vi "Main.vi"() -> ()   [LabVIEW 2011]
uses:
  2-Think/2 Typedefs/Which Boat.ctl
  0x2-OCU-Think Comm/0x2 Typedefs/Waypoints List.ctl
  2-Think/2 Classes/Waypoint/Waypoint.lvclass
  0x2-OCU-Think Comm/0x2 Typedefs/Current Waypoint.ctl
  2-Think/2 Typedefs/eStopCommand.ctl
  0x2-OCU-Think Comm/0x2 Typedefs/ocuMessage.ctl
  0x2-OCU-Think Comm/0x2 Typedefs/ocuCommands.ctl
  <vilib>/Platform/TimedLoop/XDataNode/timing_clust.ctl
  <vilib>/Platform/TimedLoop/XDataNode/nitl_modes.ctl
  <vilib>/Platform/TimedLoop/XDataNode/wakeup.ctl
  <vilib>/vision/Image Controls.llb/IMAQ Image.ctl
  2-Think/2 Globals/2 Global.vi
  2-Think/2 Globals/2 Message Logger.vi
  <vilib>/Platform/TimedLoop/XDataNode/XDataNode.xnode
  <vilib>/Platform/TimedLoop/XDataNode/XDNodeRunTimeDep.lvlib
  0x2-OCU-Think Comm/0x2 Classes/NetworkStreams/Writer/NetworkStreamWriter.lvclass
  0x2-OCU-Think Comm/0x2 Classes/NetworkStreams/Reader/NetworkStreamReader.lvclass
  2-Think/2 Classes/Logger/Logger.lvclass
panel:
  in  "Enable logging?":bool
  in  "Data storage folder":path
  in  "Which Boat Am I?":T1=enum."Simulation"
  out "E-stop freq.":dbl
  out "Act freq.":dbl
  out "Sense freq.":dbl
  out "Think freq.":dbl
  in  "E-Stop":bool
  # "this is the parent VI under which \nSense Think and Act run."
  # "Will save to U:\\Logs when run on the RIO"
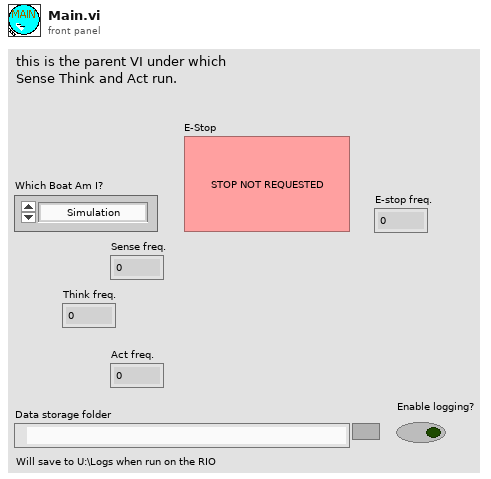
[diagram p1: front panel]
types:
  T1 = typedef "Which Boat.ctl" = enum16{"Competition Boat", "Small RC", "Simulation"}
  T2 = typedef "Waypoints List.ctl" = refnum<class "Waypoint.lvclass">[]
  T3 = typedef "Current Waypoint.ctl" = i32
  T4 = typedef "eStopCommand.ctl" = enum16{"Reset E-Stop", "Get E-Stop", "Set E-Stop"}
  T5 = typedef "ocuMessage.ctl" = cluster{"OCU Command":T6, "Data":variant}
  T6 = typedef "ocuCommands.ctl" = enum16{"Pass", "Send override", "Add waypoint", "Delete waypoint", "Set waypoint number", "Stop", "Add Mission"}
  T7 = typedef "XDNodeRunTimeDep.lvlib/timing_clust.ctl" = cluster{"Expected End [f-1]":u64, "Actual End [f-1]":u64, "Finished Late? [f-1]":bool, "Expected End [i-1]":u64, "Actual End [i-1]":u64, "Finished Late? [i-1]":bool, "Expected Start [i]":u64, "Actual Start [i]":u64, "Expected Start [f]":u64, "Actual Start [f]":u64, "Source Name":string, "Structure Name":string, "Period":i64, "Deadline":i64, "Offset":i64, "Start":i64, "Priority":i32, "Timeout":i32, "Mode":T8, "Wakeup Reason":T9, "Error":errorcluster, "Source Type":string, "Secondary Source Type":string, "Global End Time":u64, "Global Start Time":u64, "Frame Duration":u64, "Iteration Duration":u64, "Assigned CPU":i32, "I/O Scan Engine Mode":u32}
  T8 = typedef "XDNodeRunTimeDep.lvlib/nitl_modes.ctl" = enum32{"No Change", "Process missed periods, maintain original phase", "Discard missed periods, maintain original phase", "Process missed periods, ignore original phase", "Discard missed periods, ignore original phase"}
  T9 = typedef "XDNodeRunTimeDep.lvlib/wakeup.ctl" = enum32{"Normal", "Aborted", "Asynchronous wakeup", "Timing source error", "Timed loop error", "Timeout"}
  T10 = typedef "IMAQ Image.ctl" = refnum<image>
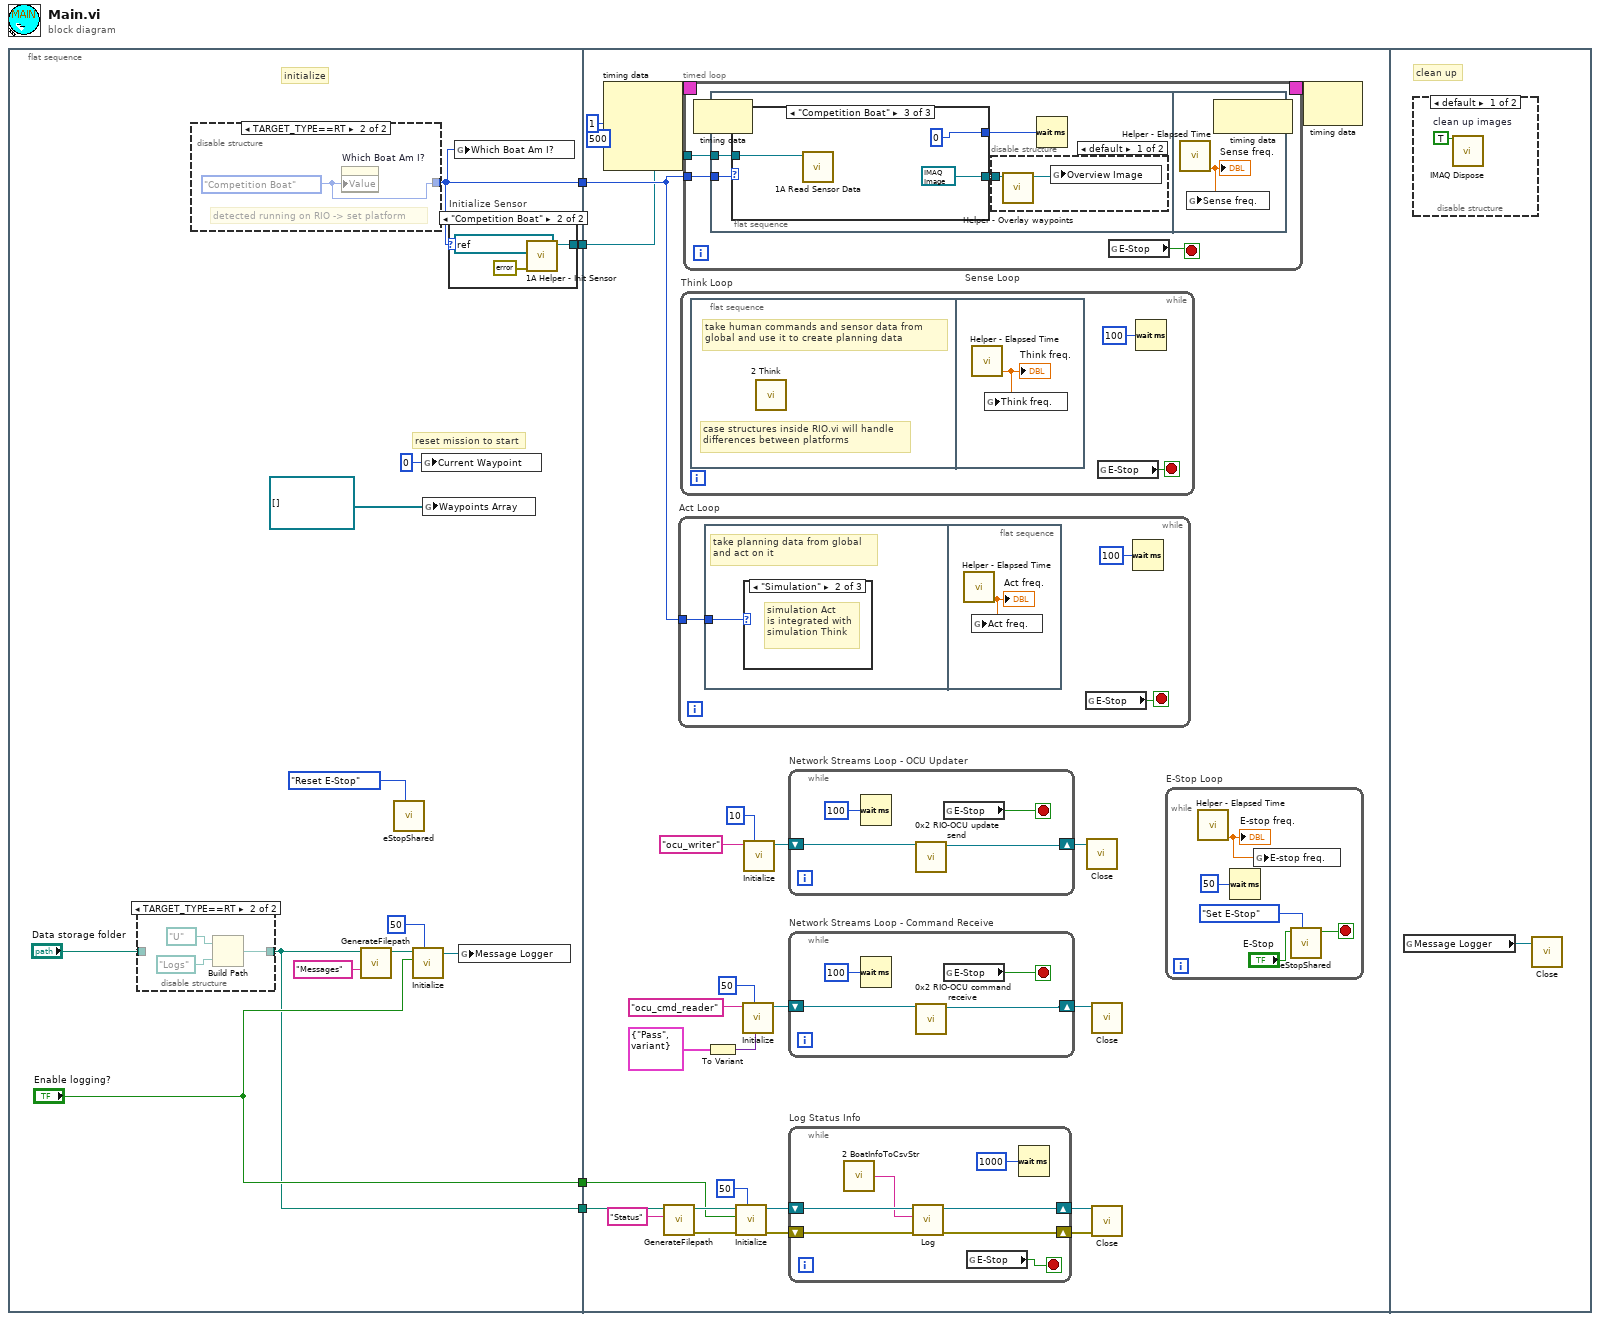
[diagram p0: block diagram]
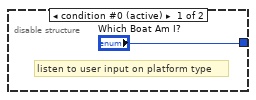
[diagram p4: hidden frame]
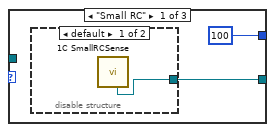
[diagram p6: hidden frame]
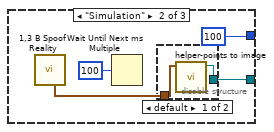
[diagram p8: hidden frame]
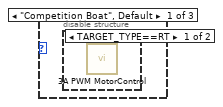
[diagram p10: hidden frame]
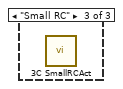
[diagram p12: hidden frame]
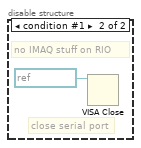
[diagram p13: hidden frame]
diagram:
  n1 = flat-sequence {
    tunnel: [w13] -> w4
    tunnel: [w14] -> w3
    tunnel: [w6] -> w2
    tunnel: ["Enable logging?"] -> w1
    tunnel: w4 -> [w51]
    tunnel: w3 -> [w50]
    tunnel: w2 -> [w30]
    tunnel: w1 -> [w26]
    frame #0 {
      # "reset mission to start"
      # "initialize"
      n2 = disable-structure shown="TARGET_TYPE==RT" {
        disable-tunnel: "Data storage folder" -> [w17 _]
        disable-tunnel: [w17 w18] -> w6
        frame condition #0 (active) {
        }
        frame condition #1 {
          n3 = Build Path(base path=path "U:/" ("Data storage folder"), name or relative path=path "Logs" ("Data storage folder")) -> (appended path=w18:path)
        }
      }
      n4 = disable-structure shown="TARGET_TYPE==RT" {
        disable-tunnel: ["Which Boat Am I?" w25] -> w13
        frame condition #0 (active) {
          # "listen to user input on platform type"
        }
        frame condition #1 {
          w25 = Which_Boat."Competition Boat" ("Which Boat Am I?")
          # "detected running on RIO -> set platform"
          n5 = property on="Which Boat Am I?" class="Enum (strict)"("Value"=w25) -> ()  [unwired: 2 in, 2 out]
        }
      }
      n6 = call "GenerateFilepath.vi"("Identifier"="Messages", "Data storage folder"=w6) -> ("File path out"=w9:path)  [unwired: 8 in, 1 out]
      n7 = call "eStopShared.vi"("Command"=eStopCommand."Reset E-Stop") -> ()  [unwired: 9 in, 2 out]
      n8 = call "Initialize.vi"("buffer size"=50, "Enable? (T)"="Enable logging?", "File path"=w9) -> ("Logger out"=w10:refnum<class "Logger.lvclass">)  [unwired: 7 in, 1 out]
      n9 = global write "2 Global.vi" "Current Waypoint"(T3 0 ("Current Waypoint")) -> ()
      n10 = global write "2 Global.vi" "Waypoints Array"(T2 [] ("Waypoints Array")) -> ()
      n11 = case "Initialize Sensor" shown="\"Competition Boat\"" w13 {
        tunnel: [_ w21] -> w14
        frame Default {
        }
        frame "Competition Boat" {
          n12 = call "1A Helper - Init Sensor.vi"("error in (no error)"=errorcluster {"status"=FALSE, "code"=0, "source"=""}, "VISA Refnum in"=refnum<visa-resource-name> "ASRL1::INSTR" ("VISA resource name")) -> ("VISA Refnum out"=w21:refnum<visa-resource-name>)  [unwired: 7 in, 2 out]
        }
      }
      n13 = global write "2 Global.vi" "Which Boat Am I?"(w13) -> ()
      n14 = global write "2 Message Logger.vi" "Message Logger"(w10) -> ()
    }
    frame #1 {
      n15 = node-c288(i64 1 ("Period"), 500 ("Priority")) -> (w49:T7)  [unwired: 2 in]
      n16 = call "GenerateFilepath.vi"("Identifier"="Status", "Data storage folder"=w30) -> ("error out"=w34:errorcluster, "File path out"=w35:path)  [unwired: 8 in]
      n17 = while "Act Loop" {
        tunnel: w51 -> [w105]
        stop <- w106 stop-if-true
        n18 = flat-sequence {
          tunnel: w105 -> [w107]
          frame #0 {
            # "take planning data from global\nand act on it"
            n19 = case shown="\"Simulation\"" w107 {
              frame "Competition Boat", Default {
                n20 = disable-structure shown="TARGET_TYPE==RT" {
                  frame condition #0 {
                    n21 = call "3A PWM MotorControl.vi"() -> ()  [unwired: 12 in]
                  }
                  frame condition #1 (active) {
                  }
                }
              }
              frame "Simulation" {
                # "simulation Act\nis integrated with\nsimulation Think"
              }
              frame "Small RC" {
                n22 = call "3C SmallRCAct.vi"() -> ()  [unwired: 12 in]
              }
            }
          }
          frame #1 {
            n23 = call "Helper - Elapsed Time.vi"() -> ("Frequency (Hz)"=w108:dbl)  [unwired: 10 in, 1 out]
            "Act freq." <- w108
            n24 = global write "2 Global.vi" "Act freq."(w108) -> ()
          }
        }
        n25 = global read "2 Global.vi" "E-Stop"() -> (w106:bool)
        n26 = Wait (ms)(milliseconds to wait=u32 100 ("millisecond multiple")) -> ()  [unwired: 1 out]
      }
      n27 = while "Think Loop" {
        stop <- w102 stop-if-true
        n28 = flat-sequence {
          frame #0 {
            # "case structures inside RIO.vi will handle\ndifferences between platforms"
            # "take human commands and sensor data from\nglobal and use it to create planning data"
            n29 = call "2 Think.vi"() -> ()  [unwired: 12 in]
          }
          frame #1 {
            n30 = call "Helper - Elapsed Time.vi"() -> ("Frequency (Hz)"=w103:dbl)  [unwired: 10 in, 1 out]
            "Think freq." <- w103
            n31 = global write "2 Global.vi" "Think freq."(w103) -> ()
          }
        }
        n32 = global read "2 Global.vi" "E-Stop"() -> (w102:bool)
        n33 = Wait (ms)(milliseconds to wait=u32 100 ("millisecond multiple")) -> ()  [unwired: 1 out]
      }
      n34 = timed-loop "Sense Loop" {
        tunnel: w51 -> [w68]
        tunnel: w50 -> [w67]
        timing: w49 -> [_]
        timing-out: [_] -> w48
        stop <- w69 stop-if-true
        n35 = node-c288() -> ()  [unwired: 1 in, 1 out]
        n36 = flat-sequence {
          tunnel: w68 -> [w74]
          tunnel: w67 -> [w72]
          frame #0 {
            n37 = case shown="\"Competition Boat\"" w74 {
              tunnel: [w79 w82 T10 refnum ("Image Out")] -> w75
              tunnel: [u32 100 ("millisecond multiple") u32 100 ("millisecond multiple") u32 0 ("millisecond multiple")] -> w73
              tunnel: w72 -> [_ _ w87]
              frame "Small RC" {
                n38 = disable-structure shown="default" {
                  disable-tunnel: [w80 _] -> w79
                  frame condition #0 (active) {
                    n39 = call "1C SmallRCSense.vi"() -> ("Eye in the Sky"=w80:T10)  [unwired: 6 in, 5 out]
                  }
                  frame condition #1 {
                  }
                }
              }
              frame "Simulation" {
                n40 = call "1,3 B Spoof Reality.vi"() -> ("Boat Path"=w83:cluster{"X Position":dbl, "Y Position":dbl}[])  [unwired: 5 in, 6 out]
                n41 = Wait Until Next ms Multiple(millisecond multiple=u32 100) -> ()  [unwired: 1 out]
                n42 = disable-structure shown="default" {
                  disable-tunnel: w83 -> [w86 _]
                  disable-tunnel: [w85 _] -> w82
                  frame condition #0 (active) {
                    n43 = call "helper-points to image.vi"("Array of Points"=w86) -> ("Image Out"=w85:T10)  [unwired: 10 in]
                  }
                  frame condition #1 {
                    # "no IMAQ\non RIO"
                  }
                }
              }
              frame "Competition Boat" {
                n44 = call "1A Read Sensor Data.vi"("VISA resource name (in)"=w87) -> ()  [unwired: 9 in, 2 out]
              }
            }
            n45 = disable-structure shown="default" {
              disable-tunnel: w75 -> [w76 _]
              frame condition #0 (active) {
                n46 = call "Helper - Overlay waypoints.vi"("Img Refnum in"=w76) -> ("Img Refnum out"=w77:T10)  [unwired: 10 in]
                n47 = global write "2 Global.vi" "Overview Image"(w77) -> ()
              }
              frame condition #1 {
                # "no IMAQ stuff on RIO"
              }
            }
            n48 = Wait (ms)(milliseconds to wait=w73) -> ()  [unwired: 1 out]
          }
          frame #1 {
            n49 = call "Helper - Elapsed Time.vi"() -> ("Frequency (Hz)"=w90:dbl)  [unwired: 10 in, 1 out]
            "Sense freq." <- w90
            n50 = global write "2 Global.vi" "Sense freq."(w90) -> ()
          }
        }
        n51 = global read "2 Global.vi" "E-Stop"() -> (w69:bool)
        n52 = node-c288() -> ()  [unwired: 1 in, 1 out]
      }
      n53 = To Variant(anything=T5 {"OCU Command"=enum."Pass", "Data"=variant} ("OCU Message")) -> (Variant=w41:variant)
      n54 = call "Initialize.vi"("buffer size"=50, "error in (no error)"=w34, "Enable? (T)"=w26, "File path"=w35) -> ("error out"=w31:errorcluster, "Logger out"=w32:refnum<class "Logger.lvclass">)  [unwired: 6 in]
      n55 = call "Initialize.vi"("Default return"=w41, "reader buffer size"=50 ("writer buffer size"), "reader name"="ocu_cmd_reader") -> ("NetworkStreamWriter out"=w37:refnum<class "NetworkStreamReader.lvclass">)  [unwired: 6 in, 2 out]
      n56 = call "Initialize.vi"("writer buffer size"=10, "writer name"="ocu_writer") -> ("NetworkStreamWriter out"=w45:refnum<class "NetworkStreamWriter.lvclass">)  [unwired: 7 in, 2 out]
      n57 = while "Network Streams Loop - OCU Updater" {
        shift-right: [w63] -> w44
        shift-left: w45 -> [w64]
        stop <- w66 stop-if-true
        n58 = Wait (ms)(milliseconds to wait=u32 100 ("millisecond multiple")) -> ()  [unwired: 1 out]
        n59 = call "0x2 RIO-OCU update send.vi"("OCU Writer In"=w64) -> ("OCU Writer Out"=w63:refnum<class "NetworkStreamWriter.lvclass">)  [unwired: 10 in]
        n60 = global read "2 Global.vi" "E-Stop"() -> (w66:bool)
      }
      n61 = while "Network Streams Loop - Command Receive" {
        shift-right: [w59] -> w38
        shift-left: w37 -> [w60]
        stop <- w62 stop-if-true
        n62 = Wait (ms)(milliseconds to wait=u32 100 ("millisecond multiple")) -> ()  [unwired: 1 out]
        n63 = call "0x2 RIO-OCU command receive.vi"("Manual Override Reader In"=w60) -> ("Manual Override Reader Out"=w59:refnum<class "NetworkStreamReader.lvclass">)  [unwired: 10 in]
        n64 = global read "2 Global.vi" "E-Stop"() -> (w62:bool)
      }
      n65 = while "Log Status Info" {
        shift-right: [w56] -> w28
        shift-left: w32 -> [w57]
        shift-right: [w55] -> w27
        shift-left: w31 -> [w54]
        stop <- w58 stop-if-true
        n66 = call "2 BoatInfoToCsvStr.vi"() -> ("CSV String"=w52:string)  [unwired: 1 in]
        n67 = call "Log.vi"("error in (no error)"=w54, "Message"=w52, "Logger in"=w57) -> ("error out"=w55:errorcluster, "Logger out"=w56:refnum<class "Logger.lvclass">)  [unwired: 7 in]
        n68 = global read "2 Global.vi" "E-Stop"() -> (w58:bool)
        n69 = Wait (ms)(milliseconds to wait=u32 1000 ("millisecond multiple")) -> ()  [unwired: 1 out]
      }
      n70 = call "Close.vi"("NetworkStreamWriter in"=w44) -> ()  [unwired: 9 in, 2 out]
      n71 = call "Close.vi"("NetworkStreamReader in"=w38) -> ()  [unwired: 9 in, 2 out]
      n72 = call "Close.vi"("error in (no error)"=w27, "NetworkStreamWriter in"=w28) -> ()  [unwired: 9 in, 1 out]
      n73 = while "E-Stop Loop" {
        stop <- w97 stop-if-true
        n74 = call "Helper - Elapsed Time.vi"() -> ("Frequency (Hz)"=w96:dbl)  [unwired: 10 in, 1 out]
        "E-stop freq." <- w96
        n75 = Wait (ms)(milliseconds to wait=u32 50 ("millisecond multiple")) -> ()  [unwired: 1 out]
        n76 = global write "2 Global.vi" "E-stop freq."(w96) -> ()
        n77 = call "eStopShared.vi"("Command"=eStopCommand."Set E-Stop", "E-Stop"="E-Stop") -> ("E-Stop Out"=w97:bool)  [unwired: 8 in, 1 out]
      }
      n78 = node-c288(w48) -> ()  [unwired: 1 out]
    }
    frame #2 {
      # "clean up"
      n79 = global read "2 Message Logger.vi" "Message Logger"() -> (w109:refnum<class "Logger.lvclass">)
      n80 = disable-structure shown="default" {
        frame condition #0 (active) {
          w110 = TRUE  # clean up images
          n81 = call "IMAQ Dispose"("All Images? (No)"=w110) -> ()  [unwired: 5 in, 1 out]
        }
        frame condition #1 {
          # "close serial port"
          # "no IMAQ stuff on RIO"
          n82 = VISA Close(VISA resource name=refnum<visa-resource-name> "COM1") -> ()  [unwired: 1 in, 1 out]
        }
      }
      n83 = call "Close.vi"("NetworkStreamWriter in"=w109) -> ()  [unwired: 10 in, 1 out]
    }
  }
